vi "Get Camera Handle.vi"(8 "error in (no error)":errorcluster, 10 "cameraHandle":i32, 11 "cameraIndex":i32) -> (0 "error out":errorcluster, 2 "cameraHandle out":i32, 3 "function return":u32)   [LabVIEW 2014, in "atmcd32d.lvlib"]
doc: "unsigned int WINAPI GetCameraHandle(long cameraIndex, long * cameraHandle);"
uses:
  atmcd32d.lvlib
  atmcd32d.dll
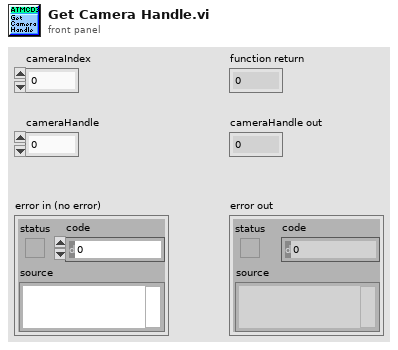
[diagram p1: front panel]
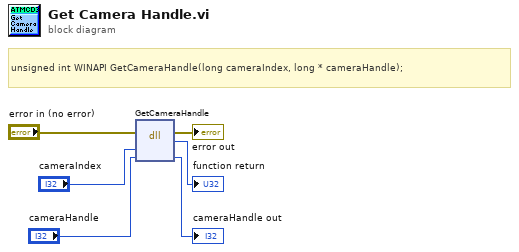
[diagram p0: block diagram]
diagram:
  # "unsigned int WINAPI GetCameraHandle(long cameraIndex, long * cameraHandle);"
  n1 = dll-call lib="C:/Users/Bakir/Documents/Lambda2-Testing/lib/Andorlib/atmcd32d.*" fn="GetCameraHandle"(error in="error in (no error)", "cameraIndex"="cameraIndex", "cameraHandle"="cameraHandle") -> (error out=→"error out":errorcluster, →"function return":u32, "cameraHandle"=→"cameraHandle out":i32)  [unwired: 3 in, 1 out]
